vi "Text to Timestamp.vi"(8 "error in (no error)":errorcluster, 9 "initial scan location":u32, 11 "Text Timestamp":string) -> (0 "error out":errorcluster, 1 "Offset Past Timestamp":u32, 2 "Local Time Offset (NaN if unspecified)":dbl, 3 "Time Stamp":timestamp format="%^<%H:%M:%S%6u\n%Y/%m/%d>T UTC")   [LabVIEW 2019, in "JDP Timestamp.lvlib"]
doc: "Supporting RFC3339, a subset of ISO8601, plus the SQLite standard formats \nRFC3339--> https://tools.ietf.org/html/rfc3339 \n Examples:\n \"2020-06-25T08:50:15.123Z\"\n \"2020-06-25T09:50:15.123+01:00\"\nSQLite Time Functions --> https://www.sqlite.org/lang_datefunc.html\n Examples:\n \"2020-06-25 08:50:15\" --> datetime() function\n\nAlso accepts reduced formats omitting some of the separators, or replacing them with spaces:\n \"2020 06 25 085015Z\""
uses:
  JDP Timestamp.lvlib
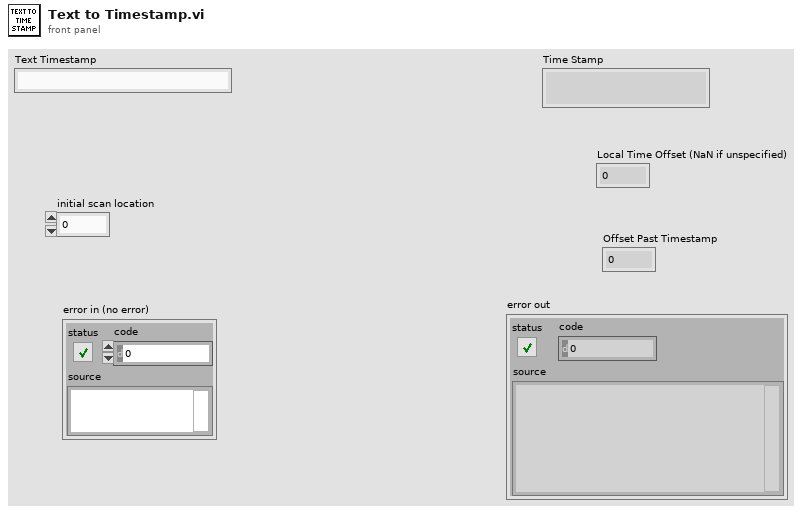
[diagram p1: front panel]
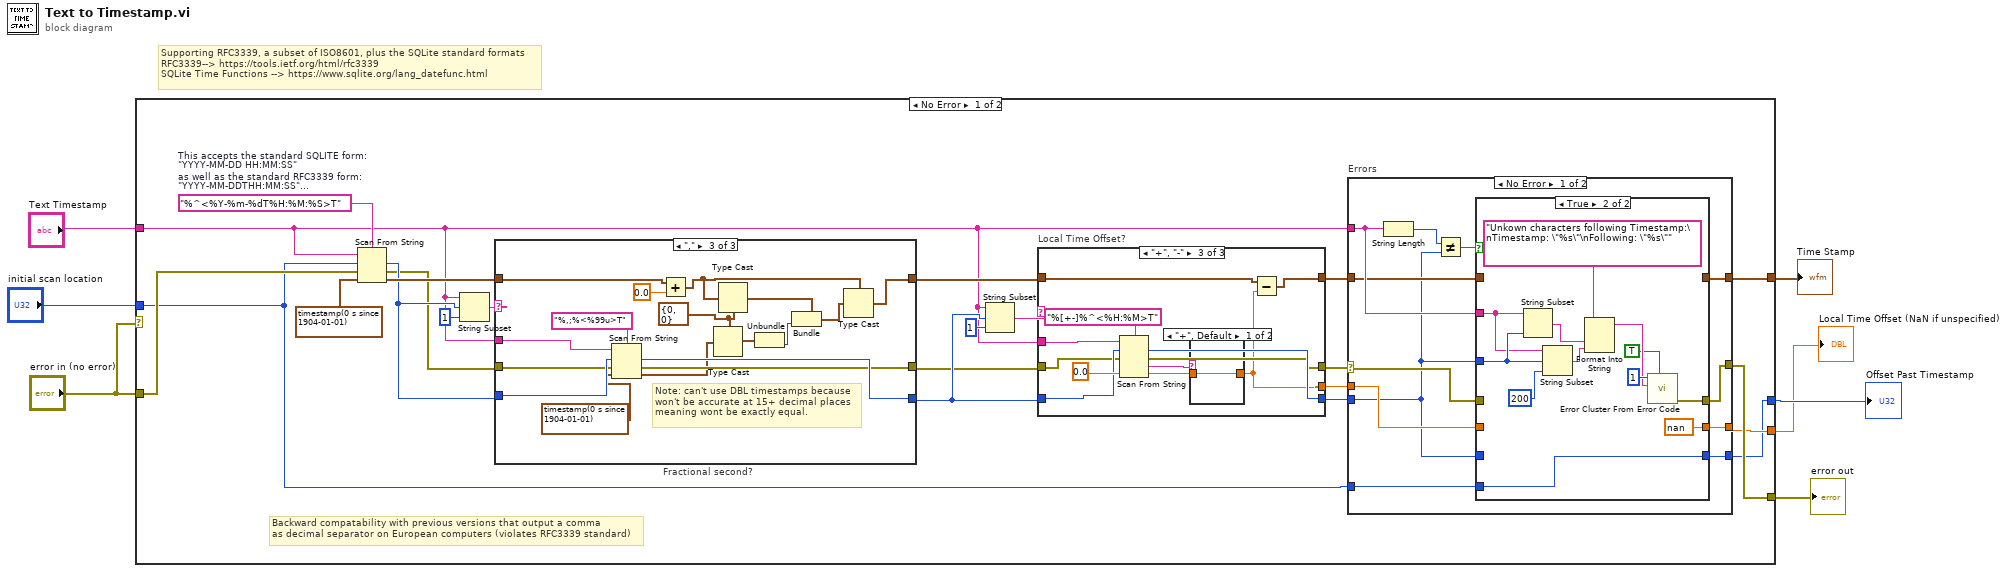
[diagram p0: block diagram]
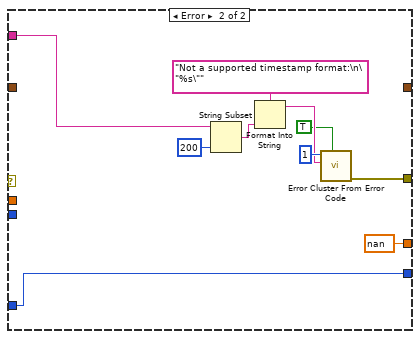
[diagram p3: hidden frame]
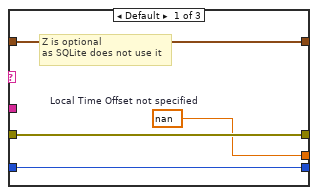
[diagram p4: hidden frame]
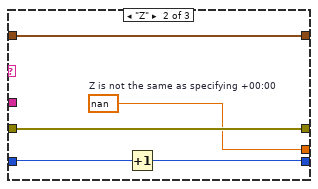
[diagram p5: hidden frame]
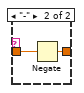
[diagram p6: hidden frame]
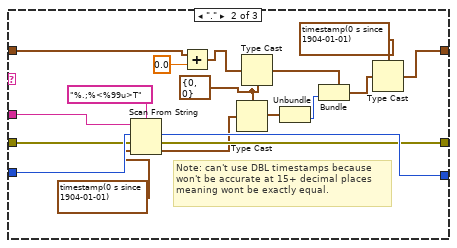
[diagram p8: hidden frame]
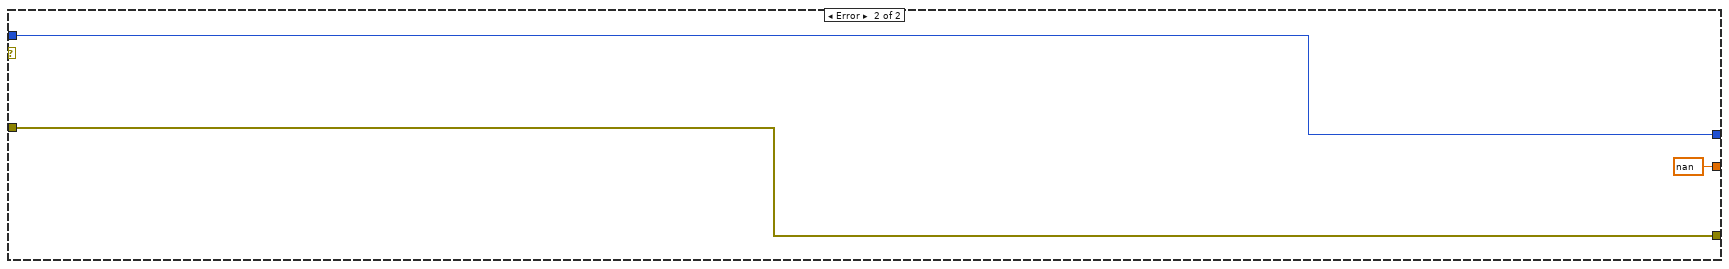
[diagram p9: hidden frame]
diagram:
  # "Supporting RFC3339, a subset of ISO8601, plus the SQLite standard formats \nRFC3339--> https://tools.ietf.org/html/rfc3339\nSQLite Time Functions --> https://www.sqlite.org/lang_datefunc.html"
  n1 = case shown="No Error" "error in (no error)" {
    tunnel: "Text Timestamp" -> [w17 _]
    tunnel: [w12 _] -> w6
    tunnel: [w9 w131] -> w5
    tunnel: "error in (no error)" -> [w20 w133]
    tunnel: [w14 w133] -> w4
    tunnel: [w10 nan] -> w2
    tunnel: "initial scan location" -> [w8 w131]
    frame No Error {
      w22 = "%^<%Y-%m-%dT%H:%M:%S>T"  # This accepts the standard SQLITE form: "YYYY-MM-DD HH:MM:SS"  as well as the standard RFC3339 form: "YYYY-MM-DDTHH:MM:SS" and ISO-8601 reduced forms that don't include some/all of the -, : or T: "YYYYMMDDHHMMSS"
      # "Backward compatability with previous versions that output a comma\nas decimal separator on European computers (violates RFC3339 standard)"
      n2 = Scan From String(format string=w22, input string=w17, initial scan location=w8, error in=w20, default 1=timestamp(0 s since 1904-01-01)) -> (offset past scan=w26:u32, error out=w19:errorcluster, output 1=w27:timestamp)  [unwired: 1 out]
      n3 = String Subset(string=w17, offset (0)=w26, length (rest)=1 ("length (rest)")) -> (substring=w28:string)
      n4 = case "Fractional second?" shown="\",\"" w28 {
        tunnel: w26 -> [w94 w110 w127]
        tunnel: w17 -> [_ w113 w130]
        tunnel: w27 -> [w95 w112 w129]
        tunnel: [w95 w111 w128] -> w25
        tunnel: [w94 w109 w126] -> w21
        tunnel: w19 -> [w93 w108 w125]
        tunnel: [w93 w107 w124] -> w18
        frame Default {
        }
        frame "." {
          w102 = cluster{i64, u64} {0, 0}
          # "Note: can't use DBL timestamps because\nwon't be accurate at 15+ decimal places\nmeaning wont be exactly equal."
          n5 = Scan From String(format string="%.;%<%99u>T", input string=w113, initial scan location=w110, error in=w108, default 1=timestamp(0 s since 1904-01-01)) -> (offset past scan=w109:u32, error out=w107:errorcluster, output 1=w103:timestamp)  [unwired: 1 out]
          n6 = Add(x=w112, y=0.0) -> (x+y=w97:timestamp)
          n7 = Type Cast(type=w102, x=w103) -> (*(type *) &x=w100:cluster{i64, u64})
          n8 = Type Cast(type=w102, x=w97) -> (*(type *) &x=w101:cluster{i64, u64})
          n9 = Unbundle(w100) -> (w99:u64)  [unwired: 1 out]
          n10 = Bundle(cluster=w101, w99) -> (w98:cluster{i64, u64})  [unwired: 1 in]
          n11 = Type Cast(type=timestamp(0 s since 1904-01-01) ("x+y"), x=w98) -> (*(type *) &x=w111:timestamp)
        }
        frame "," {
          w119 = cluster{i64, u64} {0, 0}
          # "Note: can't use DBL timestamps because\nwon't be accurate at 15+ decimal places\nmeaning wont be exactly equal."
          n12 = Scan From String(format string="%,;%<%99u>T", input string=w130, initial scan location=w127, error in=w125, default 1=timestamp(0 s since 1904-01-01)) -> (offset past scan=w126:u32, error out=w124:errorcluster, output 1=w120:timestamp)  [unwired: 1 out]
          n13 = Add(x=w129, y=0.0) -> (x+y=w114:timestamp)
          n14 = Type Cast(type=w119, x=w120) -> (*(type *) &x=w117:cluster{i64, u64})
          n15 = Type Cast(type=w119, x=w114) -> (*(type *) &x=w118:cluster{i64, u64})
          n16 = Unbundle(w117) -> (w116:u64)  [unwired: 1 out]
          n17 = Bundle(cluster=w118, w116) -> (w115:cluster{i64, u64})  [unwired: 1 in]
          n18 = Type Cast(type=w114, x=w115) -> (*(type *) &x=w128:timestamp)
        }
      }
      n19 = String Subset(string=w17, offset (0)=w21, length (rest)=1 ("length (rest)")) -> (substring=w23:string)
      n20 = case "Local Time Offset?" shown="\"+\", \"-\"" w23 {
        tunnel: w21 -> [w71 w76 w84]
        tunnel: w17 -> [_ _ w88]
        tunnel: w25 -> [w72 w77 w87]
        tunnel: [w72 w77 w85] -> w13
        tunnel: [w71 w75 w83] -> w16
        tunnel: w18 -> [w70 w74 w82]
        tunnel: [w70 w74 w81] -> w15
        tunnel: [w69 w73 w79] -> w11
        frame Default {
          w69 = nan  # Local Time Offset not specified
          # "Z is optional\nas SQLite does not use it"
        }
        frame "Z" {
          w73 = nan  # Z is not the same as specifying +00:00
          n21 = Increment(x=w76) -> (x+1=w75:u32)
        }
        frame "+", "-" {
          n22 = Scan From String(format string="%[+-]%^<%H:%M>T", input string=w88, initial scan location=w84, error in=w82, default 2=0.0) -> (offset past scan=w83:u32, error out=w81:errorcluster, output 1=w78:string, output 2=w80:dbl)  [unwired: 1 in, 1 out]
          n23 = case shown="\"+\", Default" w78 {
            tunnel: w80 -> [w90 w92]
            tunnel: [w90 w91] -> w79
            frame "+", Default {
            }
            frame "-" {
              n24 = Negate(x=w92) -> (-x=w91:dbl)
            }
          }
          n25 = Subtract(x=w87, y=w79) -> (x-y=w85:timestamp)
        }
      }
      n26 = case "Errors" shown="No Error" w15 {
        selector: w15 -> [w38 _]
        tunnel: w17 -> [w40 w66]
        tunnel: w16 -> [w32 _]
        tunnel: [w41 w61] -> w14
        tunnel: w13 -> [w36 _]
        tunnel: [w37 _] -> w12
        tunnel: w11 -> [w35 _]
        tunnel: [w34 nan] -> w10
        tunnel: [w33 w59] -> w9
        tunnel: w8 -> [w31 w59]
        frame No Error {
          n27 = String Length(string=w40) -> (length=w42:i32)
          n28 = Not Equal?(x=w42, y=w32) -> (x != y?=w39:bool)
          n29 = case shown="True" w39 {
            tunnel: [w46 w52] -> w41
            tunnel: w32 -> [_ w51]
            tunnel: w40 -> [_ w50]
            tunnel: w38 -> [w46 _]
            tunnel: [w45 _] -> w37
            tunnel: w36 -> [w45 _]
            tunnel: w35 -> [w44 _]
            tunnel: [w44 nan] -> w34
            tunnel: [w43 w47] -> w33
            tunnel: w32 -> [w43 _]
            tunnel: w31 -> [_ w47]
            frame False {
            }
            frame True {
              n30 = String Subset(string=w50, length (rest)=w51) -> (substring=w49:string)  [unwired: 1 in]
              n31 = String Subset(string=w50, offset (0)=w51, length (rest)=200 ("length (rest)")) -> (substring=w56:string)
              n32 = Format Into String(format string="Unkown characters following Timestamp:\nTimestamp: \"%s\"\nFollowing: \"%s\"", w49, w56) -> (resulting string=w54:string)  [unwired: 2 in, 1 out]
              n33 = call <vilib>:"Error Cluster From Error Code.vi"("show call chain? (False)"=TRUE, "error message (\"\")"=w54, "error code (0)"=1) -> ("error out"=w52:errorcluster)  [unwired: 6 in]
            }
          }
        }
        frame Error {
          n34 = String Subset(string=w66, length (rest)=200 ("length (rest)")) -> (substring=w65:string)  [unwired: 1 in]
          n35 = Format Into String(format string="Not a supported timestamp format:\n\"%s\"", w65) -> (resulting string=w63:string)  [unwired: 2 in, 1 out]
          n36 = call <vilib>:"Error Cluster From Error Code.vi"("show call chain? (False)"=TRUE, "error message (\"\")"=w63, "error code (0)"=1) -> ("error out"=w61:errorcluster)  [unwired: 6 in]
        }
      }
    }
    frame Error {
    }
  }
  "Time Stamp" <- w6
  "Offset Past Timestamp" <- w5
  "error out" <- w4
  "Local Time Offset (NaN if unspecified)" <- w2
